vi "Multitone Generator.vi"(4 "coerce frequencies?":bool, 5 "amplitude":dbl=-1.0 format="%.2p", 6 "sampling info":cluster{"Fs":dbl, "#s":dbl}={"Fs"=1000.0, "#s"=1000.0} {"Fs" format="%.2p"}, 7 "reset signal":bool, 8 "error in (no error)":errorcluster, 9 "tone phases":dbl[](array[numeric])=[137.63, 330.58, 66.37, 291.58] format="%.2p", 10 "tone amplitudes":dbl[](array[numeric])=[1.0, 1.0, 1.0, 1.0] format="%.2p", 11 "tone frequencies":dbl[](array[numeric])=[100.0, 200.0, 300.0, 400.0] format="%.2p") -> (0 "error out":errorcluster, 1 "actual tone frequencies":dbl[](array[numeric]), 2 "crest factor":dbl format="%.2p", 3 "signal out":waveform(dbl))   [LabVIEW 2020, in "NI_MAPro.lvlib"]
doc: "Generates a waveform that is the sum of integer cycle sine tones."
uses:
  NI_MAPro.lvlib
  NI_MABase.lvlib
  NI_AALPro.lvlib
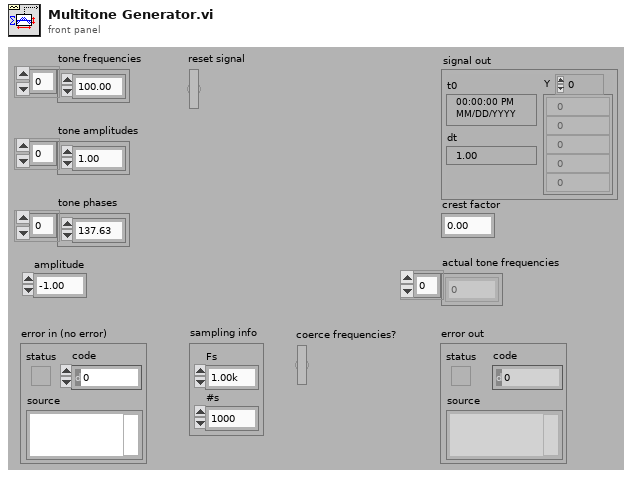
[diagram p1: front panel]
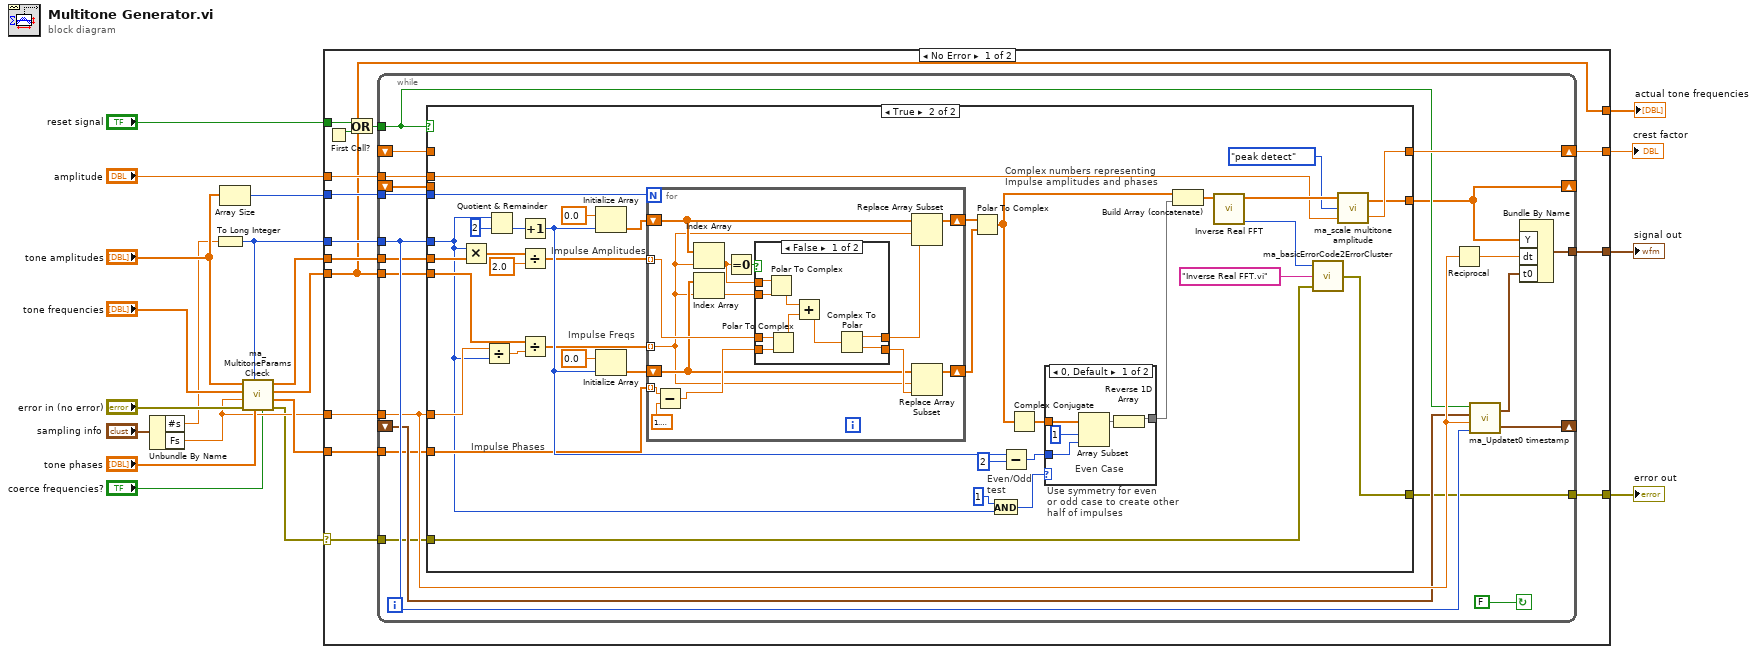
[diagram p0: block diagram]
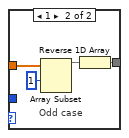
[diagram p4: hidden frame]
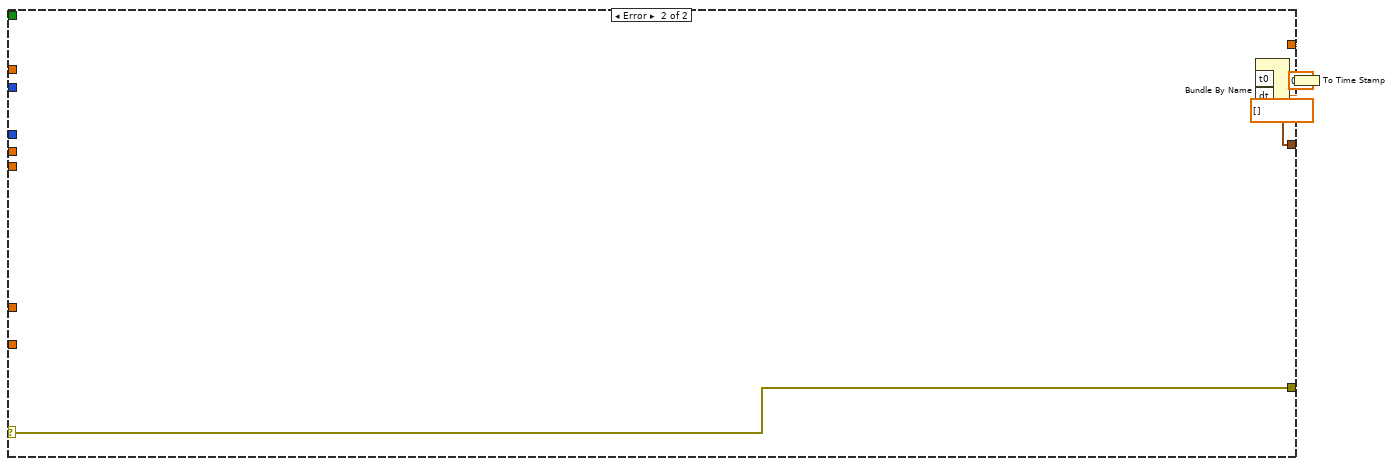
[diagram p5: hidden frame]
diagram:
  n1 = Unbundle By Name("sampling info") -> ("#s"=w9:dbl, "Fs"=w10:dbl)
  n2 = To Long Integer(number=w9) -> (32bit integer=w2:i32)
  n3 = Array Size(array="tone amplitudes") -> (size(s)=w19:i32)
  n4 = call "ma_MultitoneParamsCheck.vi"("coerce frequencies?"="coerce frequencies?", "Phases"="tone phases", "Samples"=w2, "error in (no error)"="error in (no error)", "Sampling Rate"=w10, "Tone Frequencies"="tone frequencies", "Tone Amplitudes"="tone amplitudes") -> ("error out"=w5:errorcluster, "Phases out"=w15:dbl[], "Tone Frequencies out"=w17:dbl[], "Tone Amplitudes out"=w12:dbl[])  [unwired: 1 in]
  n5 = case shown="No Error" w5 {
    selector: w5 -> [w26 w130]
    tunnel: [w34 w130] -> w20
    tunnel: w19 -> [w33 _]
    tunnel: w17 -> [w24 _]
    tunnel: w15 -> [w32 _]
    tunnel: w12 -> [w31 _]
    tunnel: w10 -> [w30 _]
    tunnel: w2 -> [w29 _]
    tunnel: "amplitude" -> [w28 _]
    tunnel: [w25 nan] -> w7
    tunnel: [w27 w132] -> w6
    tunnel: [w24 _] -> w3
    tunnel: "reset signal" -> [w21 _]
    frame No Error {
      n6 = First Call?() -> (First Call?: T/F=w23:bool)
      n7 = Or(x=w21, y=w23) -> (x .or. y?=w22:bool)
      n8 = while {
        shift-left: _ -> [w52]
        shift-right: [w41] -> _
        shift-left: _ -> [w42]
        shift-right: [w43] -> w25
        shift-left: _ -> [w44]
        shift-right: [w38] -> _
        tunnel: w22 -> [w40]
        tunnel: w26 -> [w46]
        tunnel: [w37] -> w27
        tunnel: w28 -> [w47]
        tunnel: w29 -> [w54]
        tunnel: w30 -> [w53]
        tunnel: w31 -> [w48]
        tunnel: w32 -> [w49]
        tunnel: w24 -> [w50]
        tunnel: w33 -> [w36]
        tunnel: [w51] -> w34
        stop <- FALSE continue-if-true
        n9 = case shown="True" w40 {
          tunnel: w53 -> [_ w93]
          tunnel: [w55 w94] -> w51
          tunnel: w36 -> [_ w70]
          tunnel: w54 -> [_ w61]
          tunnel: w50 -> [_ w92]
          tunnel: w49 -> [_ w67]
          tunnel: w48 -> [_ w78]
          tunnel: w47 -> [_ w64]
          tunnel: [w56 w63] -> w43
          tunnel: w46 -> [w55 w75]
          tunnel: [w57 w62] -> w38
          tunnel: w44 -> [w57 _]
          tunnel: w42 -> [w56 _]
          frame False {
          }
          frame True {
            # "Impulse Phases"
            # "Use symmetry for even\nor odd case to create other\nhalf of impulses"
            # "Even/Odd\ntest"
            # "Complex numbers representing \nImpulse amplitudes and phases"
            # "Impulse Freqs"
            # "Impulse Amplitudes"
            n10 = Multiply(x=w61, y=w78) -> (x*y=w89:dbl[])
            n11 = Divide(x=w93, y=w61) -> (x/y=w88:dbl)
            n12 = Quotient & Remainder(x=w61, y=2) -> (floor(x/y)=w59:i32)  [unwired: 1 out]
            n13 = Increment(x=w59) -> (x+1=w76:i32)
            n14 = Divide(x=w89, y=2.0) -> (x/y=w69:dbl[])
            n15 = Divide(x=w92, y=w88) -> (x/y=w68:dbl[])
            n16 = Initialize Array(0.0 ("Element Data"), w76) -> (w71:dbl[])
            n17 = Initialize Array(0.0 ("Element Data"), w76) -> (w72:dbl[])
            n18 = for {
              N: w70 -> [_]
              tunnel: w68 -> [w96] mode=indexing
              tunnel: w69 -> [w102] mode=indexing
              shift-right: [w108] -> w74
              shift-left: w71 -> [w104]
              shift-right: [w107] -> w73
              shift-left: w72 -> [w97]
              tunnel: w67 -> [w106] mode=indexing
              n19 = Subtract(x=w106, y=1.5707963267948966) -> (x-y=w101:dbl)
              n20 = Index Array(array=w104, index=w96) -> (element=w98:dbl)
              n21 = Index Array(array=w97, index=w96) -> (element=w95:dbl)
              n22 = Equal To 0?(x=w98) -> (x = 0?=w103:bool)
              n23 = case shown="False" w103 {
                tunnel: w102 -> [w115 w119]
                tunnel: w101 -> [w114 w118]
                tunnel: [w110 w119] -> w100
                tunnel: [w109 w118] -> w99
                tunnel: w98 -> [w117 _]
                tunnel: w95 -> [w116 _]
                frame False {
                  n24 = Polar To Complex(1:w116, 2:w117) -> (0:w113:cdb)
                  n25 = Polar To Complex(1:w114, 2:w115) -> (0:w112:cdb)
                  n26 = Add(x=w113, y=w112) -> (x+y=w111:cdb)
                  n27 = Complex To Polar(r * e^(i*theta)=w111) -> (r=w110:dbl, theta=w109:dbl)
                }
                frame True {
                }
              }
              n28 = Replace Array Subset(array=w104, new element=w100, index=w96) -> (w108:dbl[])
              n29 = Replace Array Subset(array=w97, new element=w99, index=w96) -> (w107:dbl[])
            }
            n30 = Polar To Complex(1:w73, 2:w74) -> (0:w85:cdb[])
            n31 = And(x=1, y=w61) -> (x .and. y?=w84:i32)
            n32 = Subtract(x=w76, y=2) -> (x-y=w77:i32)
            n33 = Complex Conjugate(1:w85) -> (0:w83:cdb[])
            n34 = case shown="0, Default" w84 {
              tunnel: [w124 w125] -> w81
              tunnel: w83 -> [w123 w128]
              tunnel: w77 -> [w120 _]
              frame 0, Default {
                # "Even Case"
                n35 = Array Subset(array=w123, index=1 ("Array Index"), length=w120) -> (w122:cdb[])
                n36 = Reverse 1D Array(array=w122) -> (reversed array=w124:cdb[])
              }
              frame 1 {
                # "Odd case"
                n37 = Array Subset(array=w128, index=1 ("Array Index")) -> (w126:cdb[])  [unwired: 1 in]
                n38 = Reverse 1D Array(array=w126) -> (reversed array=w125:cdb[])
              }
            }
            n39 = Build Array (concatenate)(w85, w81) -> (w82:cdb[])
            n40 = call "Inverse Real FFT.vi"("FFT {X}"=w82) -> ("error"=w80:i32, "X"=w66:dbl[])  [unwired: 9 in]
            n41 = call "ma_basicErrorCode2ErrorCluster.vi"("error in (no error)"=w75, "subVI name"="Inverse Real FFT.vi" ("subVI Name"), "Error Code"=w80) -> ("error out"=w94:errorcluster)
            n42 = call "ma_scale multitone amplitude.vi"("amplitude"=w64, "scaling method"=enum16{"max absolute value", "peak detect"}."peak detect", "multitone in"=w66) -> ("crest factor"=w63:dbl, "multitoneout"=w62:dbl[])
          }
        }
        n43 = Reciprocal(x=w53) -> (1/x=w39:dbl)
        n44 = call "ma_Updatet0 timestamp.vi"("samples"=w54, "sampling rate (S/s)"=w53, "tf previous"=w52, "Reset Generation"=w40) -> ("tf new"=w41:timestamp, "t0"=w35:timestamp)
        n45 = Bundle By Name("Y"=w38, "dt"=w39, "t0"=w35) -> (w37:waveform(dbl))  [unwired: 1 out]
      }
    }
    frame Error {
      w134 = 0.0 ("t0")
      n46 = To Time Stamp(1:w134) -> (0:w129:timestamp)
      n47 = Bundle By Name("t0"=w129, "dt"=w134, "Y"=dbl[] []) -> (w132:waveform(dbl))  [unwired: 1 out]
    }
  }
  "error out" <- w20
  "signal out" <- w6
  "crest factor" <- w7
  "actual tone frequencies" <- w3
